vi "port_timeouterror.vi"(8 "error in (no error)":errorcluster) -> (0 "error out":errorcluster)   [LabVIEW 2024]
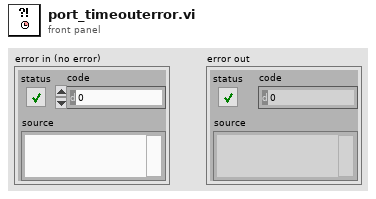
[diagram p1: front panel]
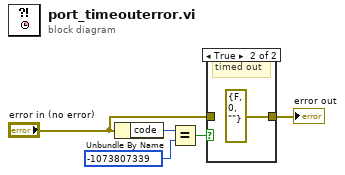
[diagram p0: block diagram]
diagram:
  n1 = Unbundle By Name("error in (no error)") -> ("code"=w1:i32)
  n2 = Equal?(x=w1, y=-1073807339 ("code")) -> (x = y?=w3:bool)
  n3 = case shown="True" w3 {
    tunnel: [w6 errorcluster {"status"=FALSE, "code"=0, "source"=""} ("error out")] -> w4
    tunnel: "error in (no error)" -> [w6 _]
    frame False {
    }
    frame True {
      # "timed out"
    }
  }
  "error out" <- w4
